vi "test_MonoMoveAndGetFilterWheelPosition.vi"(0 "device selection":enum16{"monochromator", "CCD", "SCD"}(ring), 1 "Test should pass":bool=TRUE, 5 "set-up a connection":bool=TRUE, 9 "tear down connection":bool=TRUE, 11 "error in":errorcluster, 12 "Delay between send and receive [ms]":i32=100, 13 "wait for procedure to be finished [ms]":i32=3000) -> (10 "log-file path":path, 15 "error out":errorcluster)   [LabVIEW 2023]
uses:
  Classes/Mono/Monochromator.lvclass
  <vilib>/addons/_JKI Toolkits/Caraya/classes/Assert/Assert Equal Value and Type_Variant.vi
  <vilib>/addons/_JKI Toolkits/Caraya/classes/Assert/Assert Not Error.vi
  <vilib>/addons/_JKI Toolkits/Caraya/classes/Test/Test.lvclass
  <vilib>/addons/_JKI Toolkits/Caraya/classes/Assert/Assert.lvclass
  <vilib>/Hampel Software Engineering/HSE Logger/hse-logger.lvlib
panel:
  # "Connector Pane"
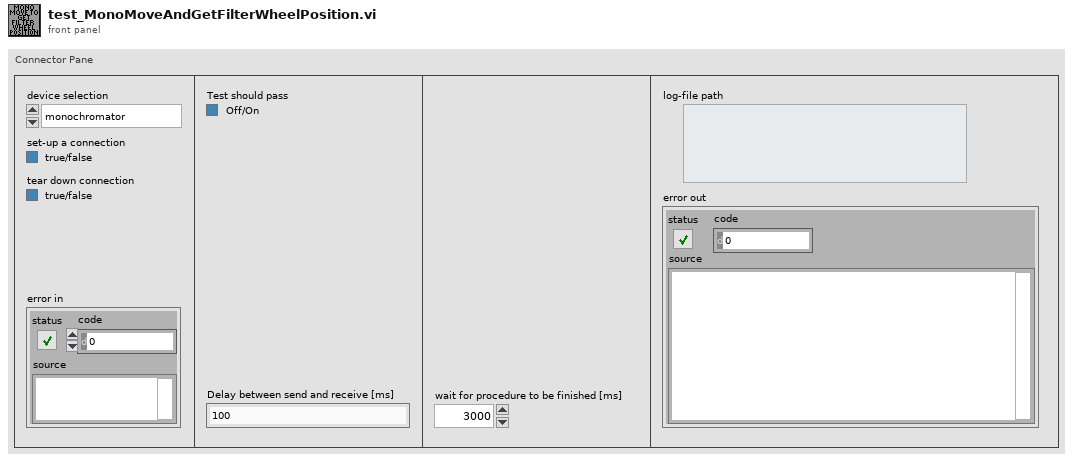
[diagram p1: front panel]
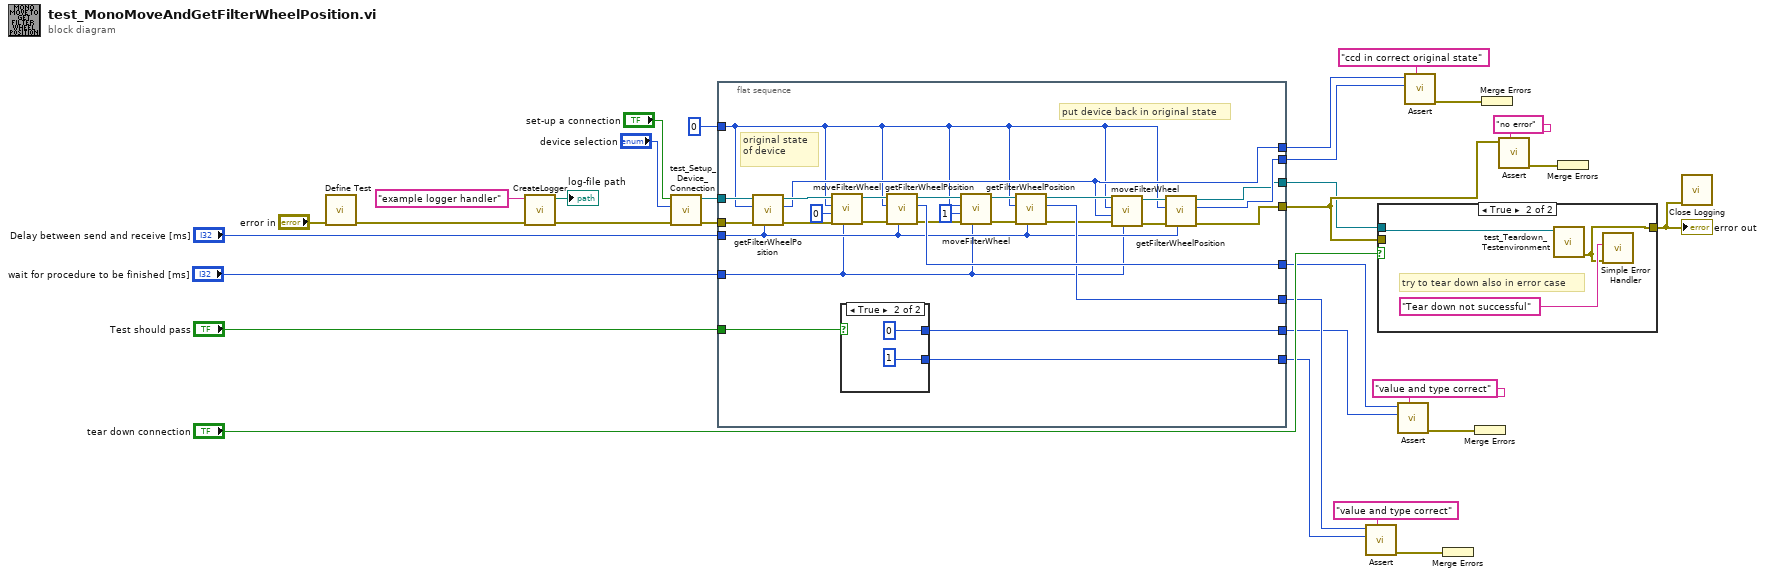
[diagram p0: block diagram]
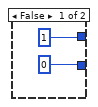
[diagram p2: hidden frame]
diagram:
  n1 = call <vilib>:"Define Test.vi"("error in (no error)"="error in") -> ("error out"=w4:errorcluster)  [unwired: 9 in, 1 out]
  n2 = call "CreateLogger.vi"("error in (no error)"=w4, "Handler Name"="example logger handler") -> ("error out"=w3:errorcluster, "log-file path"=→"log-file path":path)  [unwired: 8 in]
  n3 = call "test_Setup_Device_Connection.vi"("error in (no error)"=w3, "device selection"="device selection", "set-up a connection"="set-up a connection") -> ("error out"=w10:errorcluster, "Monochromator.lvclass"=w8:refnum<class "Monochromator.lvclass">)  [unwired: 5 in, 2 out]
  n4 = flat-sequence {
    tunnel: w10 -> [w55]
    tunnel: w8 -> [w56]
    tunnel: [w38] -> w22
    tunnel: "Test should pass" -> [w59]
    tunnel: [w39] -> w21
    tunnel: [w45] -> w20
    tunnel: [w58] -> w19
    tunnel: [w50] -> w18
    tunnel: [w57] -> w17
    tunnel: [w35] -> w14
    tunnel: [w40] -> w13
    tunnel: "Delay between send and receive [ms]" -> [w37]
    tunnel: "wait for procedure to be finished [ms]" -> [w36]
    tunnel: 0 ("type") -> [w33]
    frame #0 {
      # "put device back in original state"
      # "original state of device"
      n5 = call "getFilterWheelPosition.vi"("Delay between send and receive [ms]"=w37, "error in (no error)"=w55, "type"=w33, "Monochromator in"=w56) -> ("error out"=w53:errorcluster, "position"=w35:i32, "Monochromator out"=w54:refnum<class "Monochromator.lvclass">)  [unwired: 5 in]
      n6 = call "moveFilterWheel.vi"("Delay between send and receive [ms]"=w36, "error in (no error)"=w53, "position"=0, "type"=w33, "Monochromator in"=w54) -> ("error out"=w52:errorcluster, "Monochromator out"=w51:refnum<class "Monochromator.lvclass">)  [unwired: 3 in, 2 out]
      n7 = case shown="True" w59 {
        tunnel: [0 ("position") 1 ("position")] -> w58
        tunnel: [1 ("position") 0 ("position")] -> w57
        frame False {
        }
        frame True {
        }
      }
      n8 = call "getFilterWheelPosition.vi"("Delay between send and receive [ms]"=w37, "error in (no error)"=w52, "type"=w33, "Monochromator in"=w51) -> ("error out"=w46:errorcluster, "position"=w50:i32, "Monochromator out"=w47:refnum<class "Monochromator.lvclass">)  [unwired: 5 in]
      n9 = call "moveFilterWheel.vi"("Delay between send and receive [ms]"=w36, "error in (no error)"=w46, "position"=1, "type"=w33, "Monochromator in"=w47) -> ("error out"=w49:errorcluster, "Monochromator out"=w48:refnum<class "Monochromator.lvclass">)  [unwired: 3 in, 2 out]
      n10 = call "getFilterWheelPosition.vi"("Delay between send and receive [ms]"=w37, "error in (no error)"=w49, "type"=w33, "Monochromator in"=w48) -> ("error out"=w42:errorcluster, "position"=w45:i32, "Monochromator out"=w43:refnum<class "Monochromator.lvclass">)  [unwired: 5 in]
      n11 = call "moveFilterWheel.vi"("Delay between send and receive [ms]"=w36, "error in (no error)"=w42, "position"=w35, "type"=w33, "Monochromator in"=w43) -> ("error out"=w44:errorcluster, "Monochromator out"=w41:refnum<class "Monochromator.lvclass">)  [unwired: 3 in, 2 out]
      n12 = call "getFilterWheelPosition.vi"("Delay between send and receive [ms]"=w37, "error in (no error)"=w44, "type"=w33, "Monochromator in"=w41) -> ("error out"=w38:errorcluster, "position"=w40:i32, "Monochromator out"=w39:refnum<class "Monochromator.lvclass">)  [unwired: 5 in]
    }
  }
  n13 = call-poly <vilib>:"Assert.vi"("Label"="value and type correct" ("Label (VI Title)"), "Y"=w19, "X"=w20) -> ("error out"=w30:errorcluster)  [unwired: 7 in, 1 out]
  n14 = case shown="True" "tear down connection" {
    tunnel: w21 -> [_ w66]
    tunnel: [w64 w65] -> w1
    tunnel: w22 -> [w64 _]
    frame False {
    }
    frame True {
      # "try to tear down also in error case"
      n15 = call "test_Teardown_Testenvironment.vi"("GenericDevice.lvclass"=w66) -> ("error out"=w65:errorcluster)  [unwired: 9 in, 1 out]
      n16 = call <vilib>:"Simple Error Handler.vi"("error source (\" \")"="Tear down not successful" ("error source (\" \")"), "error in (no error)"=w65) -> ()  [unwired: 3 in, 5 out]
    }
  }
  "error out" <- w1
  n17 = call-poly <vilib>:"Assert.vi"("Label"="value and type correct" ("Label (VI Title)"), "Y"=w17, "X"=w18) -> ("error out"=w29:errorcluster)  [unwired: 7 in, 1 out]
  n18 = call-poly <vilib>:"Assert.vi"("Label"="ccd in correct original state" ("Label (VI Title)"), "Y"=w13, "X"=w14) -> ("error out"=w16:errorcluster)  [unwired: 7 in, 1 out]
  n19 = Merge Errors(w30) -> ()  [unwired: 1 out]
  n20 = Merge Errors(w29) -> ()  [unwired: 1 out]
  n21 = Merge Errors(w16) -> ()  [unwired: 1 out]
  n22 = call-poly <vilib>:"Assert.vi"("Label"="no error" ("Label (VI Title)"), "Not Error?"=w22) -> ("error out"=w24:errorcluster)  [unwired: 8 in, 1 out]
  n23 = Merge Errors(w24) -> ()  [unwired: 1 out]
  n24 = call <vilib>:"Close Logging.vi"("error in"=w1) -> ()  [unwired: 10 in, 1 out]
